vi "ACS712.vi"(11 "ACS712":dbl[](array[numeric]) format="%0.2f") -> (3 "Current":dbl)   [LabVIEW 2013, in "Test_Libraries.lvlib"]
uses:
  Proyecto/Test_Libraries.lvlib
  <vilib>/Analysis/NI_AALBase.lvlib
  <vilib>/Analysis/baseanly.llb/Mean (DBL).vi
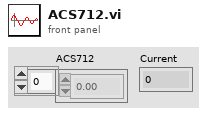
[diagram p1: front panel]
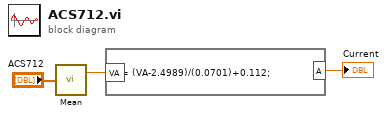
[diagram p0: block diagram]
diagram:
  n1 = call-poly <vilib>:"Mean.vi"("X"="ACS712") -> ("mean"=w3:dbl)  [unwired: 1 out]
  n2 = formula code="A= (VA-2.4989)/(0.0701)+0.112;"("VA"=w3) -> ("A"=→"Current":dbl)
